vi "ajusteNano.vi"(10 "y":dbl, 11 "x":dbl) -> ()   [LabVIEW 2018]
panel:
  in  "ajustar":bool
  in  "stop":bool
  in  "z":dbl
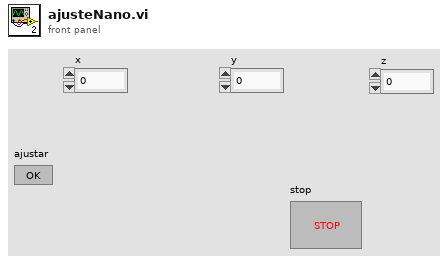
[diagram p1: front panel]
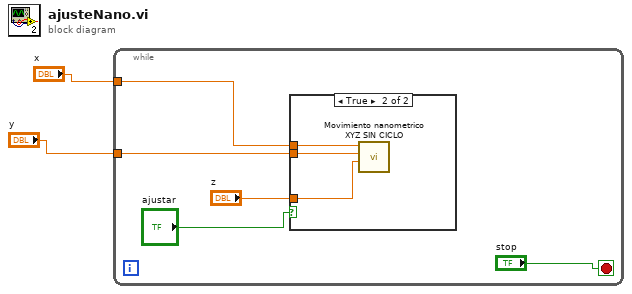
[diagram p0: block diagram]
diagram:
  n1 = while {
    tunnel: "x" -> [w6]
    tunnel: "y" -> [w5]
    stop <- "stop" stop-if-true
    n2 = case shown="True" "ajustar" {
      tunnel: w6 -> [_ w10]
      tunnel: w5 -> [_ w9]
      tunnel: "z" -> [_ w8]
      frame False {
      }
      frame True {
        n3 = call "Movimiento nanometrico XYZ SIN CICLO.vi"("Movimiento en Z"=w8, "Movimiento en Y"=w9, "Movimiento en X"=w10) -> ()  [unwired: 3 in, 1 out]
      }
    }
  }
